vi "Main.vi"(8 "error in (no error)":errorcluster, 11 "Waveform in":refnum<class "Waveform.lvclass">) -> (0 "error out":errorcluster, 3 "component":refnum<class "Waveform.lvclass">)   [LabVIEW 2012, in "Waveform.lvclass"]
doc: "Main VI of the component. This should contain the GUI of your component and be called when creating an executable."
uses:
  Waveform.lvclass
  Waveform.lvclass/Waveform.ctl
  <vilib>/Distrio/Murmex/InitialiseMessage/InitialiseMessage.lvclass
  <vilib>/Distrio/Murmex/Murmex/update_cluster.ctl
  <vilib>/Distrio/Murmex/ConfigureMessage/ConfigureMessage.lvclass
  <vilib>/Distrio/Murmex/StopMessage/StopMessage.lvclass
  <vilib>/Distrio/Murmex/StartMessage/StartMessage.lvclass
  <vilib>/Distrio/Murmex/StartMessage/run mode enum.ctl
  <vilib>/Distrio/Murmex/TerminateMessage/TerminateMessage.lvclass
  <vilib>/Distrio/Murmex/Murmex/Set configure at initialise.vi
  <vilib>/Distrio/Murmex/Murmex/Set VI reference.vi
  <vilib>/Distrio/Murmex/Murmex/Get ID.vi
  <vilib>/Distrio/Murmex/Murmex/Set relay start stop to observers.vi
  <vilib>/Distrio/Murmex/Murmex/Set log reference.vi
  <vilib>/Distrio/Murmex/Murmex/Set license required.vi
  <vilib>/Distrio/Murmex/Murmex/Set write log to disk.vi
  <vilib>/Distrio/Murmex/StartMessage/Set run mode.vi
  <vilib>/Distrio/Murmex/Murmex/Murmex.lvclass
panel:
  out "terminate?":bool=TRUE
  in  "button::quit":bool
  in  "button:start_finite":bool
  in  "button:start_free-run":bool
  in  "button::configure":bool
  in  "Tab Control":enum32{"Waveforms", "Debug"}(tab)
  in  "Delay 2":dbl[unit] caption="delay" step=1e-06
  in  "Offset 2":dbl[unit] caption="offset" min=-5.0 max=5.0 step=0.01
  in  "Amplitude 2":dbl[unit]=1.0 caption="amplitude" min=0.0 max=5.0 step=0.01
  in  "Delay 1":dbl[unit] caption="delay" step=1e-06
  in  "Offset 1":dbl[unit] caption="offset" min=-5.0 max=5.0 step=0.01
  in  "Amplitude 1":dbl[unit]=1.0 caption="amplitude" min=0.0 max=5.0 step=0.01
  out "Counter2":dbl[unit]
  out "Counter1":dbl[unit]
  in  "ID":string="waveform"
  out "HSYNC pulses":i32=2048 min=4 max=2048 step=4
  out "frame rate":dbl[unit]=100.0
  out "Mixed Signal Graph":T1(graph)
  out "log":string
  # "galvo 1"
  # "galvo 2"
  # "actual frequencies"
  # "Orca"
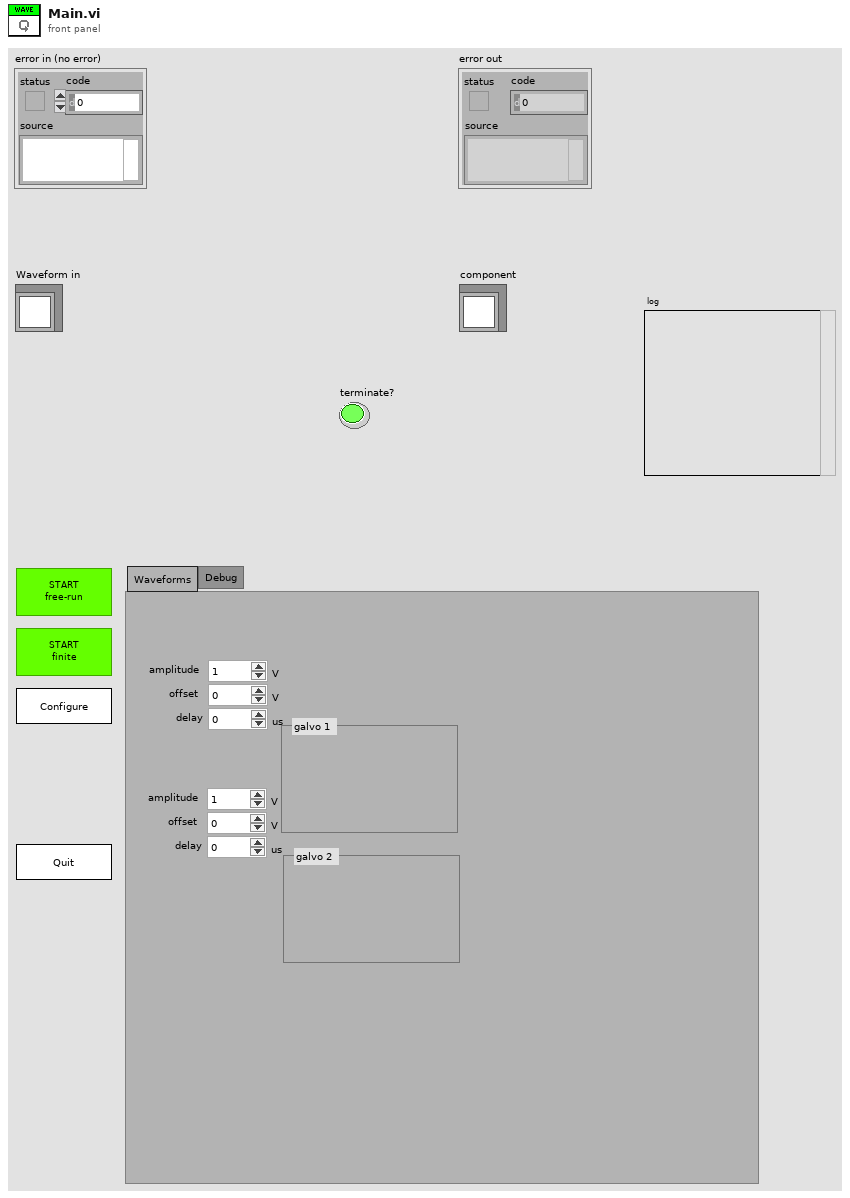
[diagram p1: front panel]
types:
  T1 = cluster{"galvo1 waveform":waveform(dbl), "galvo2 waveform":waveform(dbl), dbl[]}
  T2 = typedef "Murmex.lvlib/Murmex.lvclass/update_cluster.ctl" = cluster{"target ID":string, "key chains":string[], "values":variant[]}
  T3 = typedef "Murmex.lvlib/StartMessage.lvclass/run mode enum.ctl" = enum16{"infinite", "finite"}
  T4 = enum8{"Enabled", "Disabled", "Disabled and Grayed Out"}
  T5 = typedef "Murmex.lvlib/Murmex.lvclass/command_enum.ctl" = enum16{"null", "initialise", "reset", "terminate", "acknowledge", "update", "inspect", "inform", "proceed", "start", "stop", "fetch", "configure", "generic"}
  T6 = typedef "Murmex.lvlib/Murmex.lvclass/Event type enumerations.ctl" = enum16{"before", "after"}
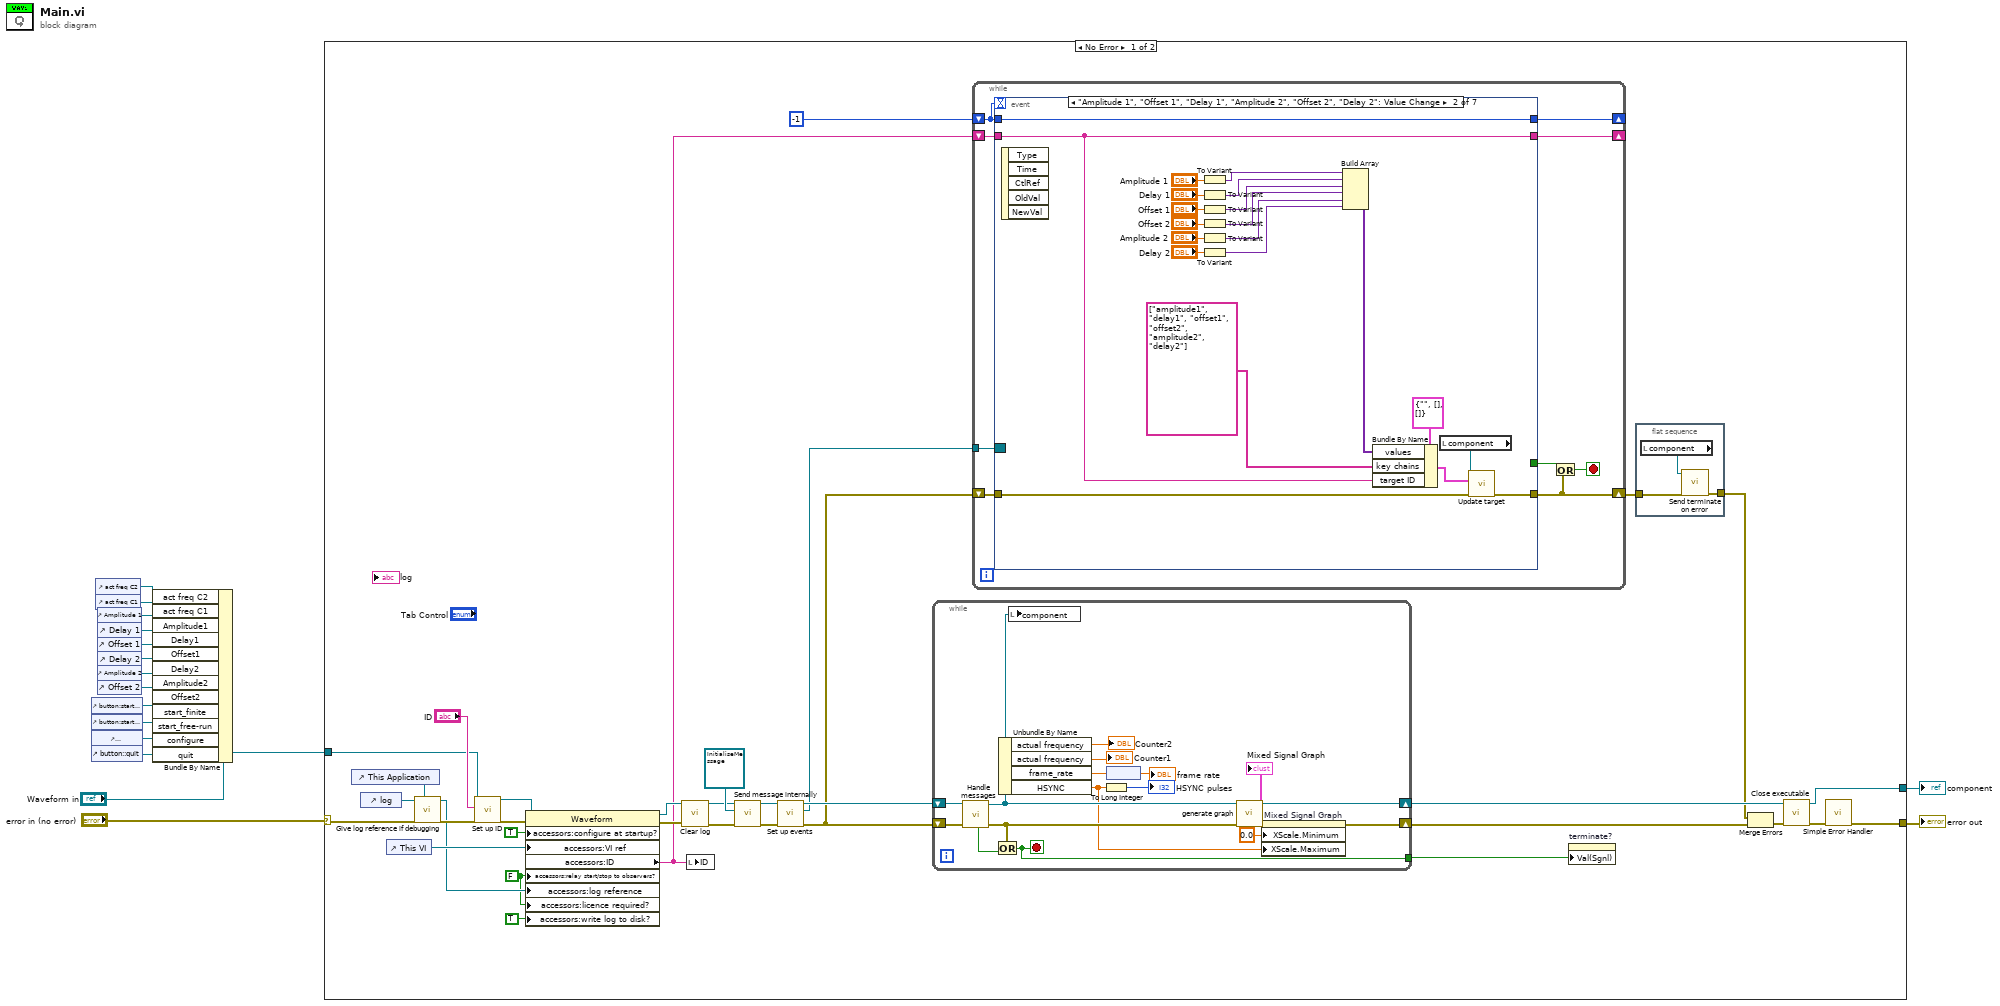
[diagram p0: block diagram]
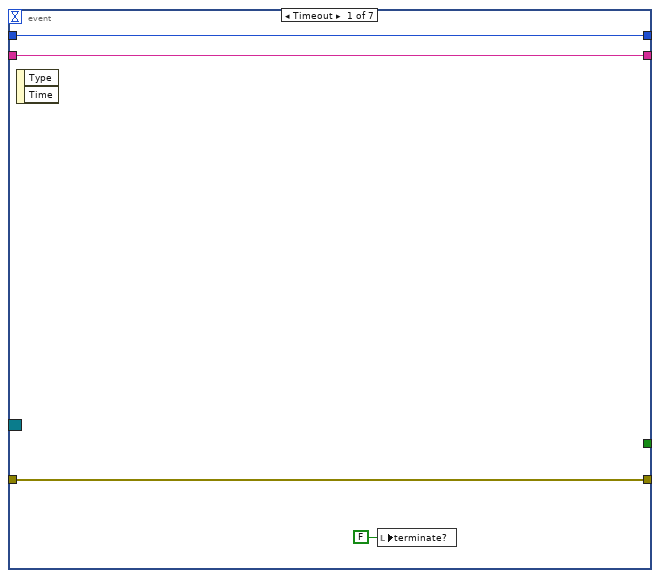
[diagram p2: hidden frame]
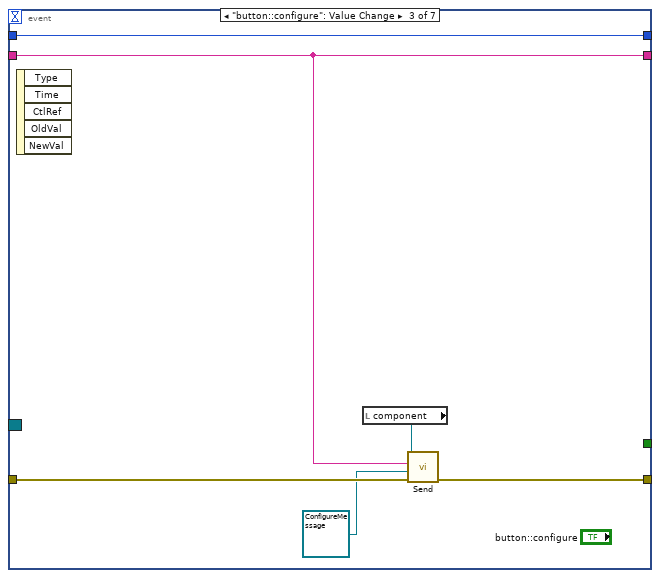
[diagram p3: hidden frame]
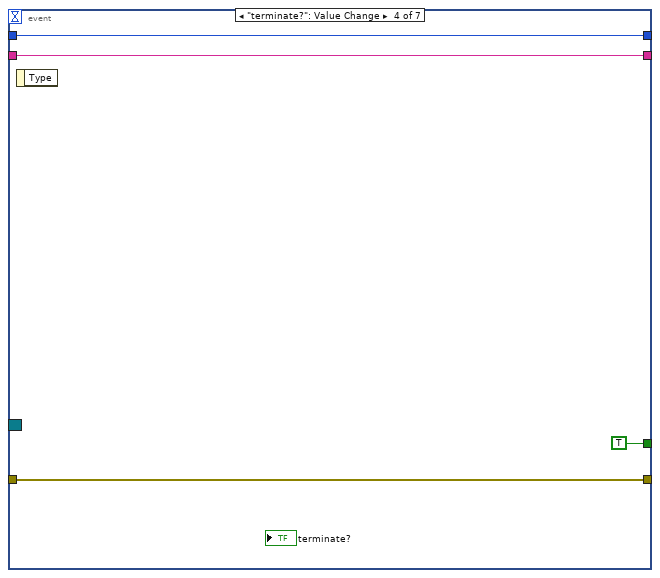
[diagram p4: hidden frame]
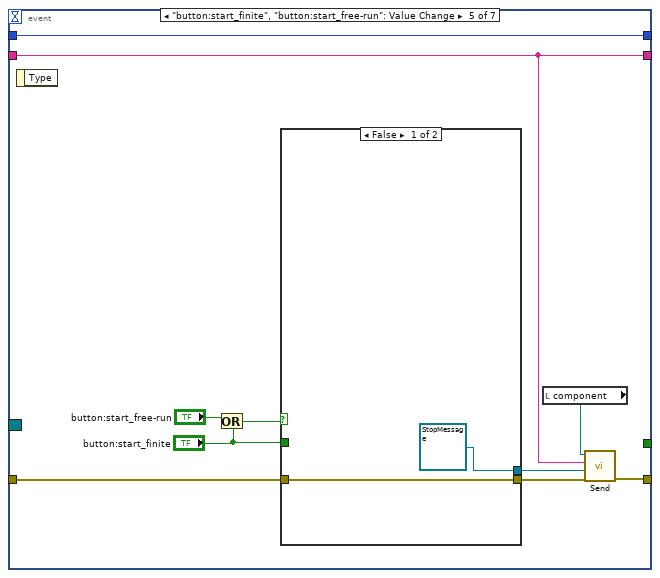
[diagram p5: hidden frame]
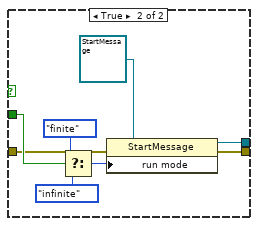
[diagram p6: hidden frame]
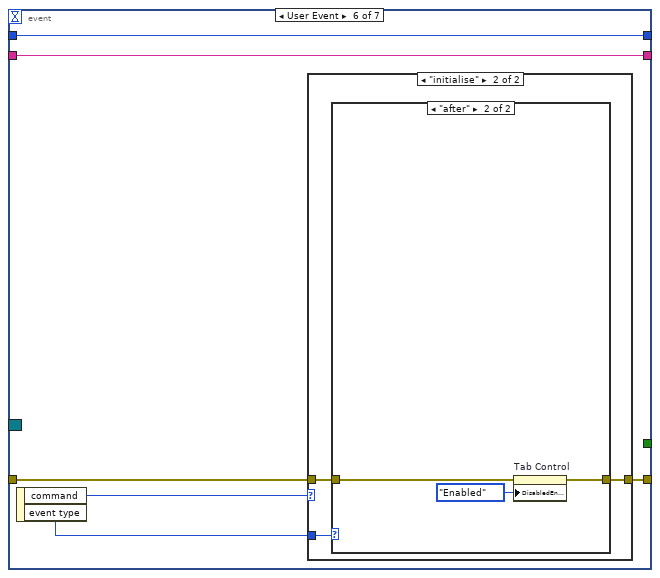
[diagram p7: hidden frame]
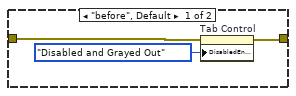
[diagram p9: hidden frame]
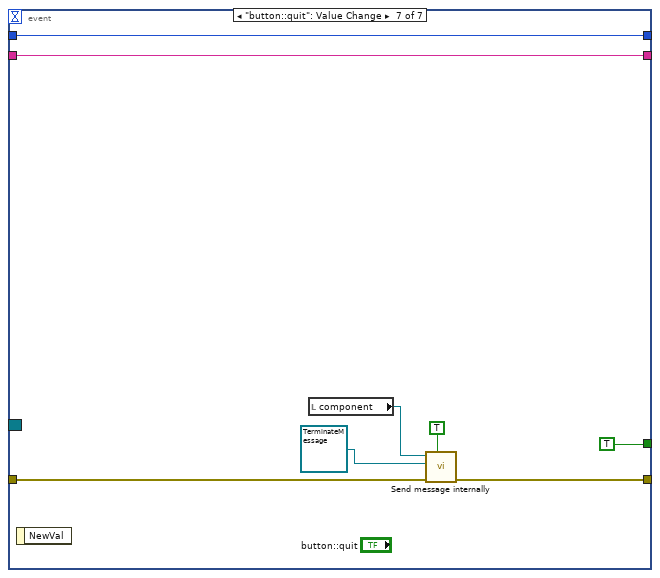
[diagram p10: hidden frame]
diagram:
  n1 = control-ref of="button:start_finite"() -> (w9:refnum<vi>)
  n2 = control-ref of="button:start_free-run"() -> (w10:refnum<vi>)
  n3 = control-ref of="button::configure"() -> (w11:refnum<vi>)
  n4 = control-ref of="button::quit"() -> (w12:refnum<vi>)
  n5 = control-ref of="act freq C2"() -> (w1:refnum<vi>)
  n6 = control-ref of="act freq C1"() -> (w2:refnum<vi>)
  n7 = control-ref of="Amplitude 1"() -> (w3:refnum<vi>)
  n8 = control-ref of="Delay 1"() -> (w4:refnum<vi>)
  n9 = control-ref of="Offset 1"() -> (w5:refnum<vi>)
  n10 = control-ref of="Delay 2"() -> (w6:refnum<vi>)
  n11 = control-ref of="Amplitude 2"() -> (w7:refnum<vi>)
  n12 = control-ref of="Offset 2"() -> (w8:refnum<vi>)
  n13 = Bundle By Name(cluster="Waveform in", "act freq C2"=w1, "act freq C1"=w2, "Amplitude1"=w3, "Delay1"=w4, "Offset1"=w5, "Delay2"=w6, "Amplitude2"=w7, "Offset2"=w8, "start_finite"=w9, "start_free-run"=w10, "configure"=w11, "quit"=w12) -> (w15:refnum<class "Waveform.lvclass">)
  n14 = case shown="No Error" "error in (no error)" {
    selector: "error in (no error)" -> [w49 w161]
    tunnel: w15 -> [w46 w160]
    tunnel: [w27 w161] -> w14
    tunnel: [w26 w160] -> w13
    frame No Error {
      w40 = FALSE ("relay start/stop to observers?")
      n15 = control-ref of="This Application"() -> (w51:refnum<vi>)
      n16 = control-ref of="log"() -> (w50:refnum<vi>)
      n17 = control-ref of="This VI"() -> (w42:refnum<vi>)
      n18 = call "Give log reference if debugging.vi"("application ref"=w51, "error in (no error)"=w49, "log reference in"=w50) -> ("error out"=w48:errorcluster, "log reference out"=w41:refnum<vi>)  [unwired: 6 in, 1 out]
      n19 = call <vilib>:"Set up ID.vi"("error in (no error)"=w48, "component ID"="ID", "MurmexBase in"=w46) -> ("error out"=w45:errorcluster, "MurmexBase out"=w44:refnum<class "Waveform.lvclass">)  [unwired: 6 in, 1 out]
      n20 = property class="Waveform"(reference=w44, error in=w45, "accessors:configure at startup?"=TRUE ("configure at startup?"), "accessors:VI ref"=w42, "accessors:relay start/stop to observers?"=w40, "accessors:log reference"=w41, "accessors:licence required?"=w40, "accessors:write log to disk?"=TRUE ("write log to disk?")) -> (reference out=w32:refnum<class "Waveform.lvclass">, error out=w33:errorcluster, "accessors:ID"=w21:string)
      n21 = call <vilib>:"Clear log.vi"("error in (no error)"=w33, "MurmexBase in"=w32) -> ("error out"=w34:errorcluster, "MurmexBase out"=w35:refnum<class "Waveform.lvclass">)  [unwired: 8 in]
      n22 = local write "ID"(w21) -> ()
      n23 = call <vilib>:"Send message internally.vi"("error in (no error)"=w34, "Message"=refnum<class "InitialiseMessage.lvclass"> refnum ("Murmex.lvlib:InitialiseMessage"), "Murmex in"=w35) -> ("error out"=w37:errorcluster, "Murmex out"=w38:refnum<class "Waveform.lvclass">)  [unwired: 7 in]
      n24 = call <vilib>:"Set up events.vi"("error in (no error)"=w37, "MurmexBase in"=w38) -> ("error out"=w23:errorcluster, "Event Registration Refnum"=w22:refnum<event-registration>, "MurmexBase out"=w31:refnum<class "Waveform.lvclass">)  [unwired: 7 in]
      n25 = while {
        shift-right: [w146] -> w28
        shift-left: w23 -> [w159]
        shift-right: [w151] -> w25
        shift-left: w31 -> [w158]
        tunnel: [w154] -> w18
        stop <- w154 stop-if-true
        n26 = call <vilib>:"Handle messages.vi"("error in (no error)"=w159, "Murmex in"=w158) -> ("error out"=w153:errorcluster, "Murmex out"=w152:refnum<class "Waveform.lvclass">, "terminated?"=w157:bool)  [unwired: 7 in]
        n27 = Or(x=w153, y=w157) -> (x .or. y?=w154:bool)
        n28 = Unbundle By Name(w152) -> ("actual frequency"=→"Counter2":dbl[unit], "actual frequency"=→"Counter1":dbl[unit], "frame_rate"=w156:dbl, "HSYNC"=w144:dbl)
        n29 = local write "component"(w152) -> ()
        n30 = To Long Integer(number=w144) -> (32bit integer=→"HSYNC pulses":i32)
        n31 = node(w156) -> (→"frame rate":dbl[unit])
        n32 = call-dynamic "generate graph.vi"("error in (no error)"=w153, "Waveform in"=w152) -> ("error out"=w147:errorcluster, "Mixed Signal Graph"=→"Mixed Signal Graph":T1, "Waveform out"=w151:refnum<class "Waveform.lvclass">)  [unwired: 7 in]
        n33 = property on="Mixed Signal Graph" class="MixedGraph (strict)"(error in=w147, "XScale.Minimum"=0.0 ("X Scale.Range:Minimum"), "XScale.Maximum"=w144) -> (error out=w146:errorcluster)  [unwired: 1 in, 1 out]
      }
      n34 = while {
        shift-right: [w61] -> _
        shift-left: -1 -> [w63]
        shift-right: [w59] -> w20
        shift-left: w23 -> [w60]
        tunnel: w22 -> [w62]
        shift-right: [w55] -> _
        shift-left: w21 -> [w56]
        stop <- w58 stop-if-true
        n35 = event shown="[1] \"Amplitude 1\", \"Offset 1\", \"Delay 1\", \"Amplitude 2\", \"Offset 2\", \"Delay 2\": Value Change" {
          selector: w62 -> [_ _ _ _ _ _ _]
          dyn-events: _ -> [_ _ _ _ _ _ _]
          timeout: w63 -> [_ _ _ _ _ _ _]
          tunnel: w63 -> [w66 w83 w90 w98 w108 w124 w136]
          tunnel: [w66 w83 w90 w98 w108 w124 w136] -> w61
          tunnel: w60 -> [w67 w85 w94 w97 w104 w122 w141]
          tunnel: [w67 w88 w93 w97 w107 w119 w140] -> w59
          tunnel: [_ _ _ TRUE ("configure at startup?") _ _ TRUE] -> w57
          tunnel: [w65 w84 w89 w95 w105 w123 w135] -> w55
          tunnel: w56 -> [w65 w84 w89 w95 w105 w123 w135]
          event Timeout {
            n36 = event-data() -> ()  [unwired: 1 in, 2 out]
            n37 = local write "terminate?"(FALSE ("terminate?")) -> ()
          }
          event "Amplitude 1", "Offset 1", "Delay 1", "Amplitude 2", "Offset 2", "Delay 2": Value Change {
            n38 = event-data() -> ()  [unwired: 1 in, 5 out]
            n39 = To Variant(anything="Amplitude 1") -> (Variant=w73:variant)
            n40 = To Variant(anything="Delay 1") -> (Variant=w72:variant)
            n41 = To Variant(anything="Offset 1") -> (Variant=w71:variant)
            n42 = To Variant(anything="Offset 2") -> (Variant=w70:variant)
            n43 = To Variant(anything="Amplitude 2") -> (Variant=w69:variant)
            n44 = To Variant(anything="Delay 2") -> (Variant=w68:variant)
            n45 = Build Array(w73, w72, w71, w70, w69, w68) -> (w81:variant[])
            n46 = Bundle By Name(cluster=T2 {"target ID"="", "key chains"=[], "values"=[]} ("update cluster"), "values"=w81, "key chains"=string[] ["amplitude1", "delay1", "offset1", "offset2", "amplitude2", "delay2"], "target ID"=w84) -> (w86:T2)
            n47 = local read "component"() -> (w82:refnum<class "Waveform.lvclass">)
            n48 = call <vilib>:"Update target.vi"("error in (no error)"=w85, "update cluster"=w86, "MurmexBase in"=w82) -> ("error out"=w88:errorcluster)  [unwired: 7 in, 1 out]
          }
          event "button::configure": Value Change {
            n49 = event-data() -> ()  [unwired: 1 in, 5 out]
            n50 = local read "component"() -> (w92:refnum<class "Waveform.lvclass">)
            n51 = call <vilib>:"Send.vi"("error in (no error)"=w94, "Message"=refnum<class "ConfigureMessage.lvclass"> refnum ("Murmex.lvlib:ConfigureMessage"), "recipient"=w89, "Murmex in"=w92) -> ("error out"=w93:errorcluster)  [unwired: 6 in, 1 out]
          }
          event "terminate?": Value Change {
            n52 = event-data() -> ()  [unwired: 1 in, 1 out]
          }
          event "button:start_finite", "button:start_free-run": Value Change {
            n53 = event-data() -> ()  [unwired: 1 in, 1 out]
            n54 = Or(x="button:start_free-run", y="button:start_finite") -> (x .or. y?=w101:bool)
            n55 = case shown="False" w101 {
              tunnel: w104 -> [w110 w117]
              tunnel: [w110 w116] -> w103
              tunnel: [refnum<class "StopMessage.lvclass"> refnum ("Murmex.lvlib:StopMessage") w114] -> w102
              tunnel: "button:start_finite" -> [_ w118]
              frame False {
              }
              frame True {
                n56 = Select(t=run_mode_enum."finite" ("run mode"), s=w118, f=run_mode_enum."infinite" ("run mode")) -> (s? t:f=w113:T3)
                n57 = property class="StartMessage"(reference=refnum<class "StartMessage.lvclass"> refnum ("Murmex.lvlib:StartMessage"), error in=w117, "run mode"=w113) -> (reference out=w114:refnum<class "StartMessage.lvclass">, error out=w116:errorcluster)
              }
            }
            n58 = local read "component"() -> (w106:refnum<class "Waveform.lvclass">)
            n59 = call <vilib>:"Send.vi"("error in (no error)"=w103, "Message"=w102, "recipient"=w105, "Murmex in"=w106) -> ("error out"=w107:errorcluster)  [unwired: 6 in, 1 out]
          }
          event User Event {
            n60 = event-data() -> ("command"=w121:T5, "event type"=w120:T6)  [unwired: 1 in]
            n61 = case shown="\"initialise\"" w121 {
              tunnel: w122 -> [w125 w127]
              tunnel: w120 -> [_ w128]
              tunnel: [w125 w126] -> w119
              frame "null", Default {
              }
              frame "initialise" {
                n62 = case shown="\"after\"" w128 {
                  tunnel: w127 -> [w129 w134]
                  tunnel: [w130 w133] -> w126
                  frame "before", Default {
                    n63 = property on="Tab Control" class="TabCtl (strict)"(error in=w129, "DisabledEnum"=T4."Disabled and Grayed Out" ("Disabled")) -> (error out=w130:errorcluster)  [unwired: 1 in, 1 out]
                  }
                  frame "after" {
                    n64 = property on="Tab Control" class="TabCtl (strict)"(error in=w134, "DisabledEnum"=T4."Enabled" ("Disabled")) -> (error out=w133:errorcluster)  [unwired: 1 in, 1 out]
                  }
                }
              }
            }
          }
          event "button::quit": Value Change {
            n65 = event-data() -> ()  [unwired: 1 in, 1 out]
            n66 = local read "component"() -> (w139:refnum<class "Waveform.lvclass">)
            n67 = call <vilib>:"Send message internally.vi"("priority message? (F)"=TRUE, "error in (no error)"=w141, "Message"=refnum<class "TerminateMessage.lvclass"> refnum ("Murmex.lvlib:TerminateMessage"), "Murmex in"=w139) -> ("error out"=w140:errorcluster)  [unwired: 6 in, 1 out]
          }
        }
        n68 = Or(x=w57, y=w59) -> (x .or. y?=w58:bool)
      }
      n69 = property on="terminate?" class="Bool (strict)"("Val(Sgnl)"=w18) -> ()  [unwired: 2 in, 2 out]
      n70 = flat-sequence {
        tunnel: w20 -> [w54]
        tunnel: [w53] -> w19
        frame #0 {
          n71 = local read "component"() -> (w52:refnum<class "Waveform.lvclass">)
          n72 = call <vilib>:"Send terminate on error.vi"("error in (no error)"=w54, "Murmex in"=w52) -> ("error out"=w53:errorcluster)  [unwired: 8 in, 1 out]
        }
      }
      n73 = Merge Errors(w19, w28) -> (w29:errorcluster)
      n74 = call <vilib>:"Close executable.vi"("error in (no error)"=w29, "MurmexBase in"=w25) -> ("error out"=w30:errorcluster, "MurmexBase out"=w26:refnum<class "Waveform.lvclass">)  [unwired: 8 in]
      n75 = call <vilib>:"Simple Error Handler.vi"("error in (no error)"=w30) -> ("error out"=w27:errorcluster)  [unwired: 4 in, 4 out]
    }
    frame Error {
    }
  }
  "error out" <- w14
  "component" <- w13
